vi "Lockin Noise Measurement.vi"(8 "error in (no error)":errorcluster, 9 "Iterations":i32, 10 "time constant (s)":dbl format="%#_6p") -> (0 "error out":errorcluster, 2 "Noise = Volts[amps]/Sqrt(Hz)":dbl[](array[numeric]) format="%#_6p")   [LabVIEW 2016]
uses:
  <vilib>/ptbypt/NI_PtbyPt.lvlib
  src/Instrument.Lockin/Instrument.Lockin.lvclass
panel:
  out "3. <|X - <X>|>":T1(graph)
  out "2. X - <X>":T1(graph)
  in  "stop":bool
  out "1. <X>":T1(graph)
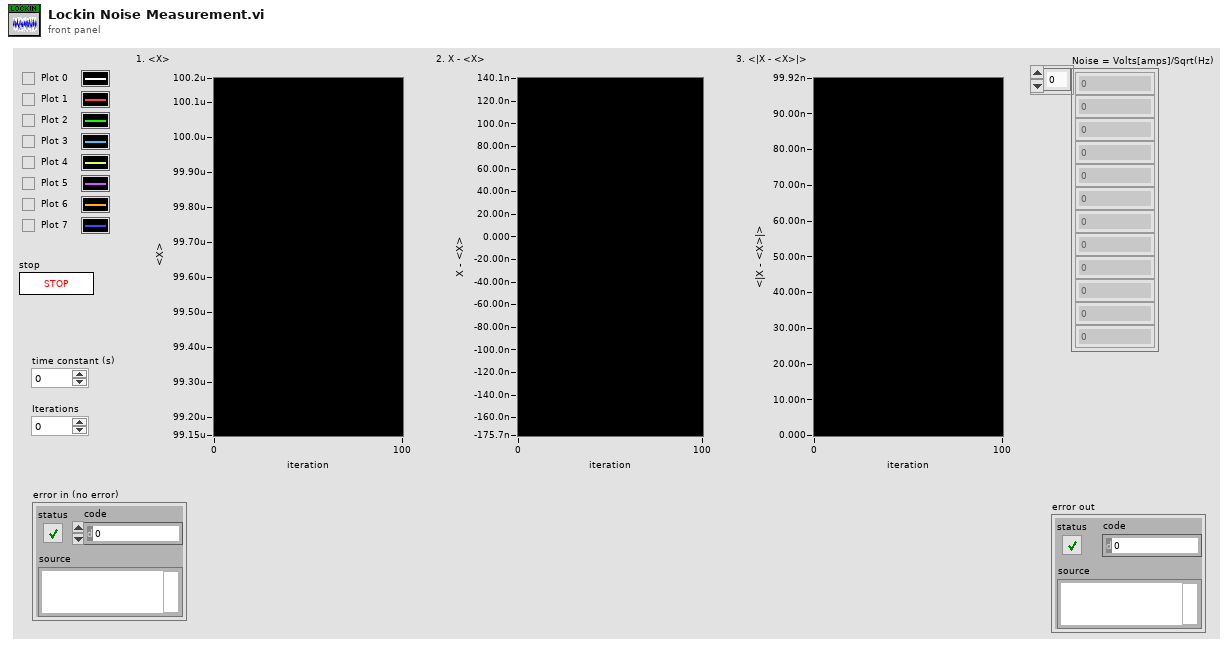
[diagram p1: front panel]
types:
  T1 = cluster{"[0]":dbl, "[1]":dbl, "[2]":dbl, "[3]":dbl, "[4]":dbl, "[5]":dbl, "[6]":dbl, "[7]":dbl, "[8]":dbl}
  T2 = cluster{"[0]":dbl, "[1]":dbl, "[2]":dbl, "[3]":dbl, "[4]":dbl, "[5]":dbl, "[6]":dbl, "[7]":dbl, "[8]":dbl}[]
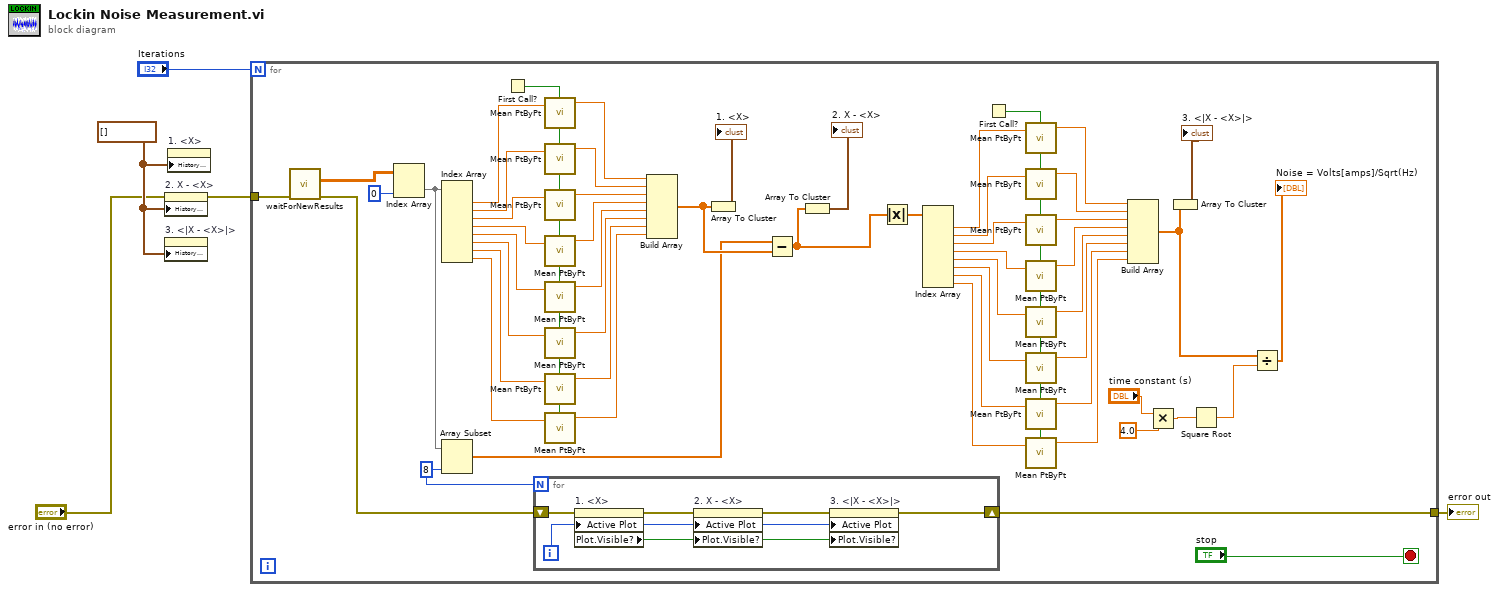
[diagram p0: block diagram]
diagram:
  w4 = T2 [] ("History Data")
  n1 = property on="2. X - <X>" class="WFChart (strict)"(error in="error in (no error)", "History Data"=w4) -> (error out=w5:errorcluster)  [unwired: 1 in, 1 out]
  n2 = property on="3. <|X - <X>|>" class="WFChart (strict)"("History Data"=w4) -> ()  [unwired: 2 in, 2 out]
  n3 = property on="1. <X>" class="WFChart (strict)"("History Data"=w4) -> ()  [unwired: 2 in, 2 out]
  n4 = for {
    N: "Iterations" -> [_]
    tunnel: w5 -> [w6]
    tunnel: [w10] -> w2
    stop <- "stop" stop-if-true
    w37 = 8 ("length")
    n5 = call "waitForNewResults.vi"("error in (no error)"=w6) -> ("error out"=w7:errorcluster, "Results"=w8:dbl[][])  [unwired: 8 in, 1 out]
    n6 = Index Array(array=w8, index (col)=0 ("disabled index (col)")) -> (element=w38:dbl[])  [unwired: 1 in]
    n7 = Index Array(array=w38) -> (element #1=w59:dbl, element #2=w58:dbl, element #3=w57:dbl, element #4=w56:dbl, element #5=w55:dbl, element #6=w54:dbl, element #7=w53:dbl, element #8=w52:dbl)  [unwired: 8 in]
    n8 = Array Subset(array=w38, length=w37) -> (w39:dbl[])  [unwired: 1 in]
    n9 = First Call?() -> (First Call?: T/F=w40:bool)
    n10 = for {
      N: w37 -> [_]
      shift-right: [w61] -> w10
      shift-left: w7 -> [w66]
      i -> [w63]
      n11 = property on="1. <X>" class="WFChart (strict)"(error in=w66, "Active Plot"=w63) -> (error out=w65:errorcluster, "Plot.Visible?"=w64:bool)  [unwired: 1 in, 1 out]
      n12 = property on="2. X - <X>" class="WFChart (strict)"(error in=w65, "Active Plot"=w63, "Plot.Visible?"=w64) -> (error out=w62:errorcluster)  [unwired: 1 in, 1 out]
      n13 = property on="3. <|X - <X>|>" class="WFChart (strict)"(error in=w62, "Active Plot"=w63, "Plot.Visible?"=w64) -> (error out=w61:errorcluster)  [unwired: 1 in, 1 out]
    }
    n14 = call <vilib>:"Mean PtByPt.vi"("x"=w59, "initialize"=w40) -> ("mean"=w51:dbl)  [unwired: 2 in, 1 out]
    n15 = call <vilib>:"Mean PtByPt.vi"("x"=w58, "initialize"=w40) -> ("mean"=w50:dbl)  [unwired: 2 in, 1 out]
    n16 = call <vilib>:"Mean PtByPt.vi"("x"=w57, "initialize"=w40) -> ("mean"=w49:dbl)  [unwired: 2 in, 1 out]
    n17 = call <vilib>:"Mean PtByPt.vi"("x"=w56, "initialize"=w40) -> ("mean"=w48:dbl)  [unwired: 2 in, 1 out]
    n18 = call <vilib>:"Mean PtByPt.vi"("x"=w55, "initialize"=w40) -> ("mean"=w47:dbl)  [unwired: 2 in, 1 out]
    n19 = call <vilib>:"Mean PtByPt.vi"("x"=w54, "initialize"=w40) -> ("mean"=w46:dbl)  [unwired: 2 in, 1 out]
    n20 = call <vilib>:"Mean PtByPt.vi"("x"=w53, "initialize"=w40) -> ("mean"=w45:dbl)  [unwired: 2 in, 1 out]
    n21 = call <vilib>:"Mean PtByPt.vi"("x"=w52, "initialize"=w40) -> ("mean"=w44:dbl)  [unwired: 2 in, 1 out]
    n22 = Build Array(w51, w50, w49, w48, w47, w46, w45, w44) -> (w42:dbl[])
    n23 = Array To Cluster(array=w42) -> (cluster=→"1. <X>":T1)
    n24 = Subtract(x=w39, y=w42) -> (x-y=w17:dbl[])
    n25 = Array To Cluster(array=w17) -> (cluster=→"2. X - <X>":T1)
    n26 = Absolute Value(x=w17) -> (abs(x)=w18:dbl[])
    n27 = Index Array(array=w18) -> (element #1=w20:dbl, element #2=w21:dbl, element #3=w22:dbl, element #4=w23:dbl, element #5=w24:dbl, element #6=w25:dbl, element #7=w26:dbl, element #8=w27:dbl)  [unwired: 8 in]
    n28 = First Call?() -> (First Call?: T/F=w36:bool)
    n29 = call <vilib>:"Mean PtByPt.vi"("x"=w20, "initialize"=w36) -> ("mean"=w28:dbl)  [unwired: 2 in, 1 out]
    n30 = call <vilib>:"Mean PtByPt.vi"("x"=w21, "initialize"=w36) -> ("mean"=w29:dbl)  [unwired: 2 in, 1 out]
    n31 = call <vilib>:"Mean PtByPt.vi"("x"=w22, "initialize"=w36) -> ("mean"=w30:dbl)  [unwired: 2 in, 1 out]
    n32 = call <vilib>:"Mean PtByPt.vi"("x"=w23, "initialize"=w36) -> ("mean"=w31:dbl)  [unwired: 2 in, 1 out]
    n33 = call <vilib>:"Mean PtByPt.vi"("x"=w24, "initialize"=w36) -> ("mean"=w32:dbl)  [unwired: 2 in, 1 out]
    n34 = call <vilib>:"Mean PtByPt.vi"("x"=w25, "initialize"=w36) -> ("mean"=w33:dbl)  [unwired: 2 in, 1 out]
    n35 = call <vilib>:"Mean PtByPt.vi"("x"=w26, "initialize"=w36) -> ("mean"=w34:dbl)  [unwired: 2 in, 1 out]
    n36 = call <vilib>:"Mean PtByPt.vi"("x"=w27, "initialize"=w36) -> ("mean"=w35:dbl)  [unwired: 2 in, 1 out]
    n37 = Build Array(w28, w29, w30, w31, w32, w33, w34, w35) -> (w16:dbl[])
    n38 = Multiply(x="time constant (s)", y=4.0) -> (x*y=w13:dbl)
    n39 = Array To Cluster(array=w16) -> (cluster=→"3. <|X - <X>|>":T1)
    n40 = Square Root(x=w13) -> (sqrt(x)=w12:dbl)
    n41 = Divide(x=w16, y=w12) -> (x/y=→"Noise = Volts[amps]/Sqrt(Hz)":dbl[])
  }
  "error out" <- w2
